vi "SimpleMove.vi"(11 "DataIn":T5) -> (3 "DataOut":T1)   [LabVIEW 2017]
doc: "SubVI criada para simular uma jogada simples do PC nas partidas Player x PC. A jogada é realizada na coordenada (*,*)."
uses:
  controls/DataIn.ctl
  controls/Tabuleiro.ctl
  controls/GameOption.ctl
  controls/Table.ctl
  controls/DataOut.ctl
  controls/TabuleiroCoordenadas.ctl
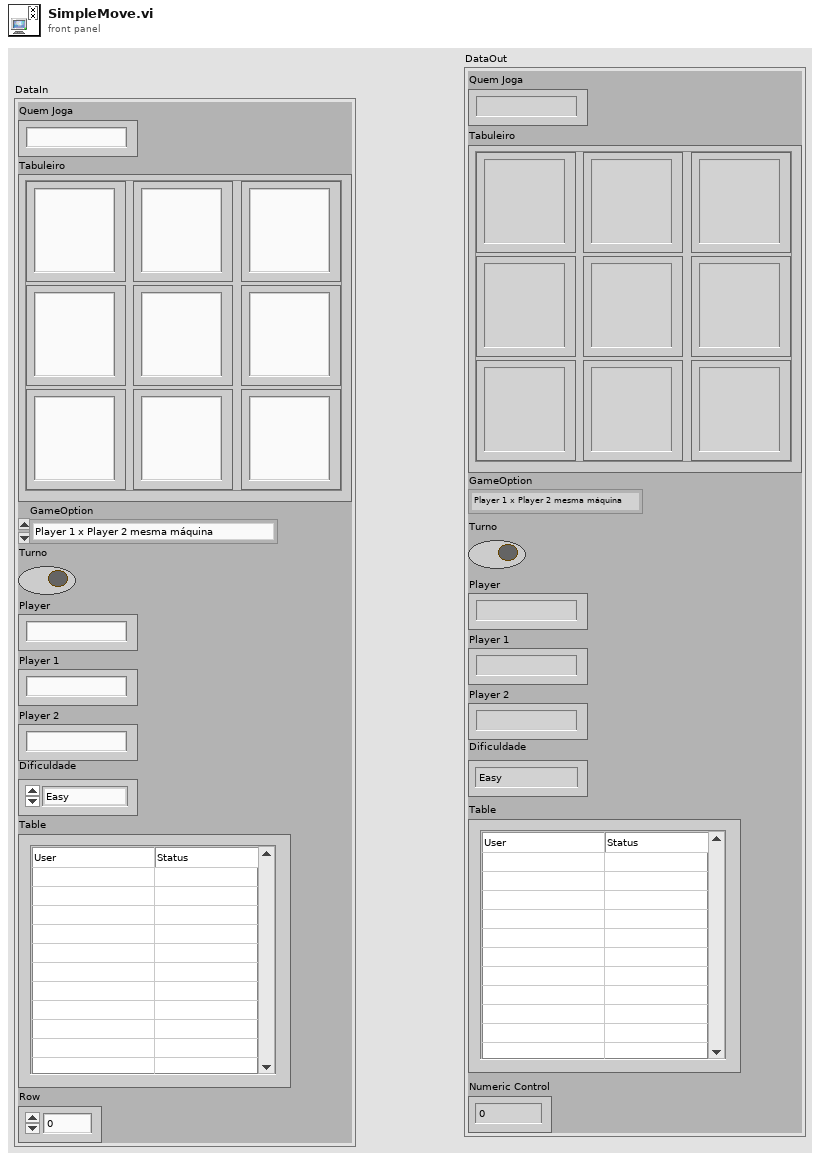
[diagram p1: front panel]
types:
  T1 = typedef "DataOut.ctl" = cluster{"Quem Joga":string, "Tabuleiro":T2, "GameOption":T3, "Turno":bool, "Player":string, "Player 1":string, "Player 2":string, "Dificuldade":enum16{"Easy", "Medium", "Hard"}, "Table":T4, "Numeric Control":u32}
  T2 = typedef "Tabuleiro.ctl" = cluster{"(0,0)":string, "(1,0)":string, "(0,1)":string, "(1,1)":string, "(2,0)":string, "(1,2)":string, "(2,2)":string, "(0,2)":string, "(2,1) ":string}
  T3 = typedef "GameOption.ctl" = enum16{"Player 1 x Player 2 mesma máquina", "Player 1 x Player 2 pela rede", "Player 1 x Computador", "Wait for Event", "Initialize", "Stop"}
  T4 = typedef "Table.ctl" = string[][]
  T5 = typedef "DataIn.ctl" = cluster{"Quem Joga":string, "Tabuleiro":T2, "GameOption":T3, "Turno":bool, "Player":string, "Player 1":string, "Player 2":string, "Dificuldade":enum16{"Easy", "Medium", "Hard"}, "Table":T4, "Row":u32}
  T6 = typedef "TabuleiroCoordenadas.ctl" = enum16{"0,0", "0,1", "0,2", "1,0", "1,1", "1,2", "2,0", "2,1", "2,2"}
  T7 = cluster{"[0]":dbl, "[1]":dbl, "[2]":dbl, "[3]":dbl, "[4]":dbl, "[5]":dbl, "[6]":dbl, "[7]":dbl, "[8]":dbl}
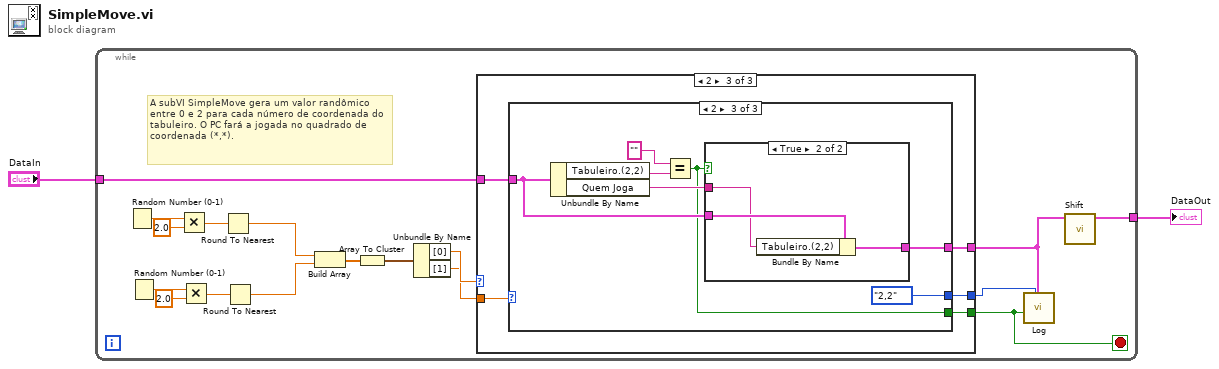
[diagram p0: block diagram]
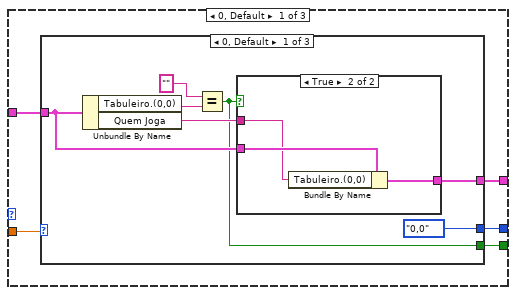
[diagram p2: hidden frame]
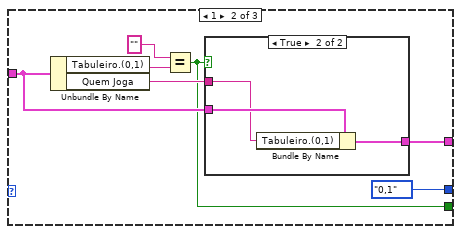
[diagram p4: hidden frame]
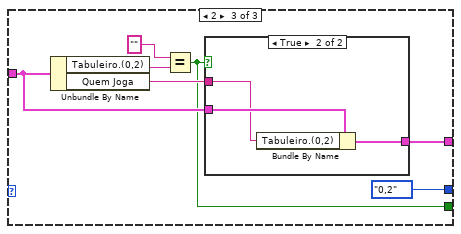
[diagram p6: hidden frame]
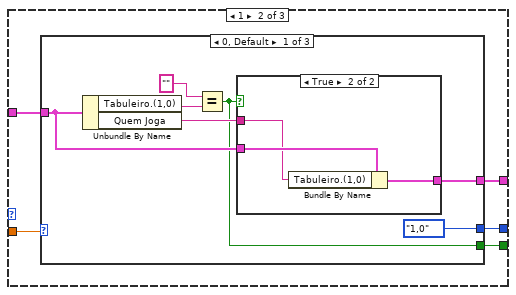
[diagram p8: hidden frame]
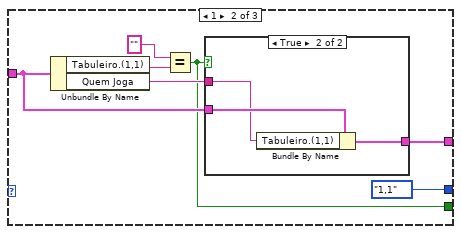
[diagram p10: hidden frame]
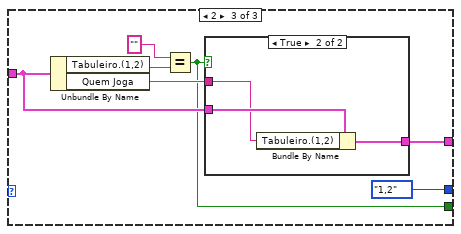
[diagram p12: hidden frame]
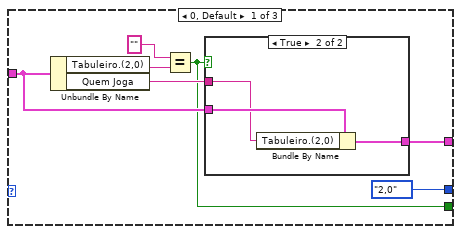
[diagram p14: hidden frame]
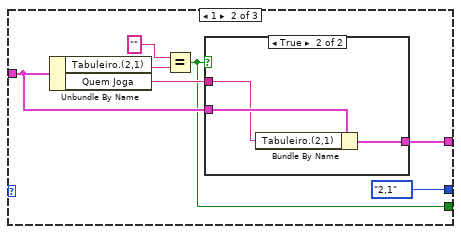
[diagram p16: hidden frame]
diagram:
  n1 = while {
    tunnel: "DataIn" -> [w7]
    tunnel: [w5] -> w1
    stop <- w3 stop-if-true
    # "A subVI SimpleMove gera um valor randômico entre 0 e 2 para cada número de coordenada do tabuleiro. O PC fará a jogada no quadrado de coordenada (*,*)."
    n2 = Random Number (0-1)() -> (number: 0 to 1=w19:dbl)
    n3 = Random Number (0-1)() -> (number: 0 to 1=w14:dbl)
    n4 = Multiply(x=w19, y=2.0) -> (x*y=w17:dbl)
    n5 = Multiply(x=w14, y=2.0) -> (x*y=w16:dbl)
    n6 = Round To Nearest(number=w17) -> (nearest integer value=w13:dbl)
    n7 = Round To Nearest(number=w16) -> (nearest integer value=w12:dbl)
    n8 = Build Array(w13, w12) -> (w11:dbl[])
    n9 = Array To Cluster(array=w11) -> (cluster=w10:T7)
    n10 = Unbundle By Name(w10) -> ("[0]"=w9:dbl, "[1]"=w8:dbl)
    n11 = case shown="2" w9 {
      tunnel: w8 -> [w23 w61 w99]
      tunnel: w7 -> [w24 w62 w100]
      tunnel: [w22 w60 w98] -> w6
      tunnel: [w21 w59 w97] -> w4
      tunnel: [w20 w58 w96] -> w3
      frame 0, Default {
        n12 = case shown="0, Default" w23 {
          tunnel: w24 -> [w28 w39 w50]
          tunnel: [w27 w38 w49] -> w22
          tunnel: [TabuleiroCoordenadas."0,0" ("Enum Coordenadas") TabuleiroCoordenadas."0,1" ("Enum Coordenadas") TabuleiroCoordenadas."0,2" ("Enum Coordenadas")] -> w21
          tunnel: [w25 w36 w47] -> w20
          frame 0, Default {
            n13 = Unbundle By Name(w28) -> ("Tabuleiro.(0,0)"=w31:string, "Quem Joga"=w29:string)
            n14 = Equal?(x="", y=w31) -> (x = y?=w25:bool)
            n15 = case shown="True" w25 {
              tunnel: w29 -> [_ w34]
              tunnel: w28 -> [w32 w35]
              tunnel: [w32 w33] -> w27
              frame False {
              }
              frame True {
                n16 = Bundle By Name(cluster=w35, "Tabuleiro.(0,0)"=w34) -> (w33:T5)
              }
            }
          }
          frame 1 {
            n17 = Unbundle By Name(w39) -> ("Tabuleiro.(0,1)"=w42:string, "Quem Joga"=w40:string)
            n18 = Equal?(x="", y=w42) -> (x = y?=w36:bool)
            n19 = case shown="True" w36 {
              tunnel: w40 -> [_ w45]
              tunnel: w39 -> [w43 w46]
              tunnel: [w43 w44] -> w38
              frame False {
              }
              frame True {
                n20 = Bundle By Name(cluster=w46, "Tabuleiro.(0,1)"=w45) -> (w44:T5)
              }
            }
          }
          frame 2 {
            n21 = Unbundle By Name(w50) -> ("Tabuleiro.(0,2)"=w53:string, "Quem Joga"=w51:string)
            n22 = Equal?(x="", y=w53) -> (x = y?=w47:bool)
            n23 = case shown="True" w47 {
              tunnel: w51 -> [_ w56]
              tunnel: w50 -> [w54 w57]
              tunnel: [w54 w55] -> w49
              frame False {
              }
              frame True {
                n24 = Bundle By Name(cluster=w57, "Tabuleiro.(0,2)"=w56) -> (w55:T5)
              }
            }
          }
        }
      }
      frame 1 {
        n25 = case shown="0, Default" w61 {
          tunnel: w62 -> [w66 w77 w88]
          tunnel: [w65 w76 w87] -> w60
          tunnel: [TabuleiroCoordenadas."1,0" ("Enum Coordenadas") TabuleiroCoordenadas."1,1" ("Enum Coordenadas") TabuleiroCoordenadas."1,2" ("Enum Coordenadas")] -> w59
          tunnel: [w63 w74 w85] -> w58
          frame 0, Default {
            n26 = Unbundle By Name(w66) -> ("Tabuleiro.(1,0)"=w69:string, "Quem Joga"=w67:string)
            n27 = Equal?(x="", y=w69) -> (x = y?=w63:bool)
            n28 = case shown="True" w63 {
              tunnel: w67 -> [_ w72]
              tunnel: w66 -> [w70 w73]
              tunnel: [w70 w71] -> w65
              frame False {
              }
              frame True {
                n29 = Bundle By Name(cluster=w73, "Tabuleiro.(1,0)"=w72) -> (w71:T5)
              }
            }
          }
          frame 1 {
            n30 = Unbundle By Name(w77) -> ("Tabuleiro.(1,1)"=w80:string, "Quem Joga"=w78:string)
            n31 = Equal?(x="", y=w80) -> (x = y?=w74:bool)
            n32 = case shown="True" w74 {
              tunnel: w78 -> [_ w83]
              tunnel: w77 -> [w81 w84]
              tunnel: [w81 w82] -> w76
              frame False {
              }
              frame True {
                n33 = Bundle By Name(cluster=w84, "Tabuleiro.(1,1)"=w83) -> (w82:T5)
              }
            }
          }
          frame 2 {
            n34 = Unbundle By Name(w88) -> ("Tabuleiro.(1,2)"=w91:string, "Quem Joga"=w89:string)
            n35 = Equal?(x="", y=w91) -> (x = y?=w85:bool)
            n36 = case shown="True" w85 {
              tunnel: w89 -> [_ w94]
              tunnel: w88 -> [w92 w95]
              tunnel: [w92 w93] -> w87
              frame False {
              }
              frame True {
                n37 = Bundle By Name(cluster=w95, "Tabuleiro.(1,2)"=w94) -> (w93:T5)
              }
            }
          }
        }
      }
      frame 2 {
        n38 = case shown="2" w99 {
          tunnel: w100 -> [w104 w115 w126]
          tunnel: [w103 w114 w125] -> w98
          tunnel: [TabuleiroCoordenadas."2,0" ("Enum Coordenadas") TabuleiroCoordenadas."2,1" ("Enum Coordenadas") TabuleiroCoordenadas."2,2" ("Enum Coordenadas")] -> w97
          tunnel: [w101 w112 w123] -> w96
          frame 0, Default {
            n39 = Unbundle By Name(w104) -> ("Tabuleiro.(2,0)"=w107:string, "Quem Joga"=w105:string)
            n40 = Equal?(x="", y=w107) -> (x = y?=w101:bool)
            n41 = case shown="True" w101 {
              tunnel: w105 -> [_ w110]
              tunnel: w104 -> [w108 w111]
              tunnel: [w108 w109] -> w103
              frame False {
              }
              frame True {
                n42 = Bundle By Name(cluster=w111, "Tabuleiro.(2,0)"=w110) -> (w109:T5)
              }
            }
          }
          frame 1 {
            n43 = Unbundle By Name(w115) -> ("Tabuleiro.(2,1)"=w118:string, "Quem Joga"=w116:string)
            n44 = Equal?(x="", y=w118) -> (x = y?=w112:bool)
            n45 = case shown="True" w112 {
              tunnel: w116 -> [_ w121]
              tunnel: w115 -> [w119 w122]
              tunnel: [w119 w120] -> w114
              frame False {
              }
              frame True {
                n46 = Bundle By Name(cluster=w122, "Tabuleiro.(2,1)"=w121) -> (w120:T5)
              }
            }
          }
          frame 2 {
            n47 = Unbundle By Name(w126) -> ("Tabuleiro.(2,2)"=w129:string, "Quem Joga"=w127:string)
            n48 = Equal?(x="", y=w129) -> (x = y?=w123:bool)
            n49 = case shown="True" w123 {
              tunnel: w127 -> [_ w132]
              tunnel: w126 -> [w130 w133]
              tunnel: [w130 w131] -> w125
              frame False {
              }
              frame True {
                n50 = Bundle By Name(cluster=w133, "Tabuleiro.(2,2)"=w132) -> (w131:T5)
              }
            }
          }
        }
      }
    }
    n51 = call "Log.vi"("Enum Coordenadas"=w4, "Confirmação"=w3, "DataIn"=w6) -> ()  [unwired: 7 in, 2 out]
    n52 = call "Shift.vi"("DataIn"=w6) -> ("DataOut"=w5:T1)  [unwired: 8 in, 2 out]
  }
  "DataOut" <- w1
